vi "Read Source Code Poll.vi"(8 "error in (no error)":errorcluster, 11 "Job Initialize in":refnum<class "Job Initialize.lvclass">) -> (0 "error out":errorcluster, 2 "Source Code Poll":T1, 3 "Job Initialize out":refnum<class "Job Initialize.lvclass">)   [LabVIEW 2014, in "Job Initialize.lvclass"]
uses:
  Job Initialize.lvclass
  Controls/Source Code Control Selection - STYP.ctl
  Job Initialize.lvclass/Job Initialize.ctl
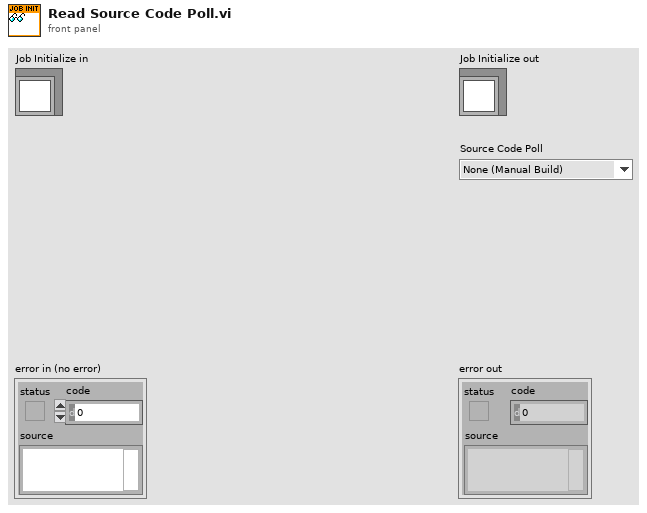
[diagram p1: front panel]
types:
  T1 = typedef "Source Code Control Selection - STYP.ctl" = enum16{"None (Manual Build)", "Every 15 Minutes", "Every 30 Minutes", "Every 45 Minutes", "Every Hour", "Every 2 Hours", "Everyday "}
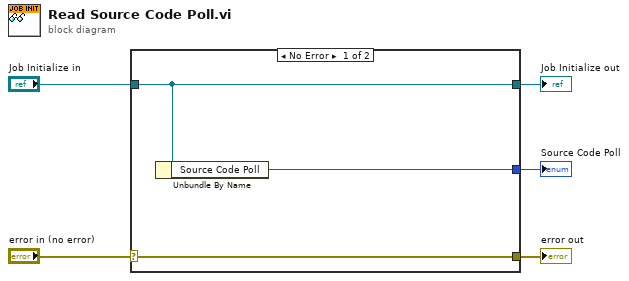
[diagram p0: block diagram]
diagram:
  n1 = case shown="No Error" "error in (no error)" {
    selector: "error in (no error)" -> [w8 w9]
    tunnel: [w8 w9] -> w4
    tunnel: [w7 w10] -> w2
    tunnel: "Job Initialize in" -> [w7 w10]
    tunnel: [w6 _] -> w1
    frame No Error {
      n2 = Unbundle By Name(w7) -> ("Source Code Poll"=w6:T1)
    }
    frame Error {
    }
  }
  "error out" <- w4
  "Job Initialize out" <- w2
  "Source Code Poll" <- w1
